vi "Get time signal.vi"(9 "init":bool, 10 "sample rate":dbl, 11 "n input samples":i32) -> (2 "t2":dbl[](array[numeric]), 3 "t":dbl[](array[numeric]))   [LabVIEW 2012]
uses:
  <vilib>/Analysis/1siggen.llb/Ramp Pattern by Samples.vi
  <vilib>/Analysis/NI_AALBase.lvlib
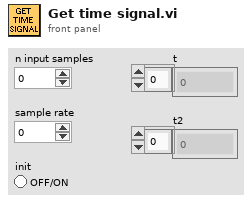
[diagram p1: front panel]
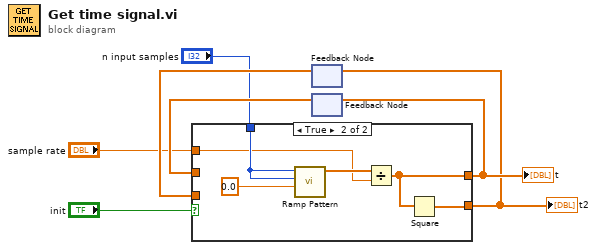
[diagram p0: block diagram]
diagram:
  n1 = feedback #1() -> (w5:dbl[])  [unwired: 1 in]
  n2 = feedback #2() -> (w4:dbl[])  [unwired: 1 in]
  n3 = case shown="True" "init" {
    tunnel: "n input samples" -> [_ w14]
    tunnel: "sample rate" -> [_ w12]
    tunnel: [w9 w11] -> w7
    tunnel: [w8 w10] -> w6
    tunnel: w4 -> [w9 _]
    tunnel: w5 -> [w8 _]
    frame False {
    }
    frame True {
      n4 = call-poly <vilib>:"Ramp Pattern.vi"("start"=0.0, "end"=w14, "samples"=w14) -> ("Ramp Pattern"=w13:dbl[])  [unwired: 7 in, 1 out]
      n5 = Divide(x=w13, y=w12) -> (x/y=w11:dbl[])
      n6 = Square(x=w11) -> (x^2=w10:dbl[])
    }
  }
  "t" <- w7
  "t2" <- w6
  n7 = feedback-in #1(w6) -> ()
  n8 = feedback-in #2(w7) -> ()
